vi "Get All Malleable VIs.vi"(8 "error in (no error)":errorcluster, 11 "VI Ref In":refnum<vi>) -> (0 "error out":errorcluster, 2 "Malleable VIs":refnum<vi>[](array[refnum]), 3 "VI Ref Out":refnum<vi>)   [LabVIEW 2020]
doc: "Searches the block diagram of the VI for any subVIs which are malleable. If none are found, Malleable VIs will be empty."
uses:
  <vilib>/Utility/traverseref.llb/TRef TravTarget.ctl
  <vilib>/Utility/traverseref.llb/VI Scripting - Traverse.lvlib
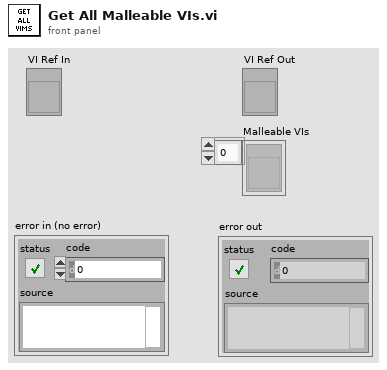
[diagram p1: front panel]
types:
  T1 = typedef "TRef TravTarget.ctl" = enum16{"FP", "BD", "Other"}
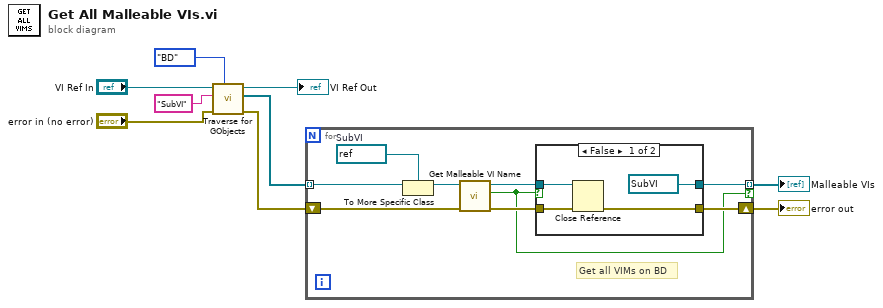
[diagram p0: block diagram]
diagram:
  n1 = call <vilib>:"Traverse for GObjects.vi"("Traverse Target"=TRef_TravTarget."BD", "error in (no error)"="error in (no error)", "Class Name"="SubVI", "VI Refnum"="VI Ref In") -> ("error out"=w2:errorcluster, "References"=w3:refnum<vi>[], "dup VI Refnum"=→"VI Ref Out":refnum<vi>)  [unwired: 4 in, 1 out]
  n2 = for {
    tunnel: w3 -> [w13] mode=indexing
    tunnel: [w14] -> w9 mode=indexing if=w10
    shift-right: [w15] -> w8
    shift-left: w2 -> [w18]
    w12 = refnum<vi> refnum  # SubVI
    # "Get all VIMs on BD"
    n3 = To More Specific Class(target class=w12, reference=w13) -> (specific class reference=w11:refnum<vi>)  [unwired: 1 in, 1 out]
    n4 = call "Get Malleable VI Name.vi"("error in (no error)"=w18, "SubVI Ref In"=w11) -> ("error out"=w16:errorcluster, "Is Malleable VI?"=w10:bool, "SubVI Ref Out"=w17:refnum<vi>)  [unwired: 5 in, 2 out]
    n5 = case shown="False" w10 {
      tunnel: w17 -> [w22 w24]
      tunnel: w16 -> [w21 w23]
      tunnel: [w20 w23] -> w15
      tunnel: [refnum<vi> refnum ("SubVI Ref Out") w24] -> w14
      frame False {
        n6 = Close Reference(reference=w22, error in (no error)=w21) -> (error out=w20:errorcluster)
      }
      frame True {
      }
    }
  }
  "Malleable VIs" <- w9
  "error out" <- w8
